vi "Test SenseHat.Actor.vi"() -> ()   [LabVIEW 2020]
uses:
  src/RPI.SenseHat.Joystick/TypeDefs/Joystick.ctl
  <vilib>/ActorFramework/Message Enqueuer/Message Enqueuer.lvclass/Message Enqueuer.ctl
  src/RPI.SenseHat.Actor/RPI.SenseHat.Actor Messages/Fill Display Msg/Fill Display Msg.lvclass/Fill Display Msg.ctl
  src/RPI.SenseHat.Actor/RPI.SenseHat.Actor Messages/Draw Display Msg/Draw Display Msg.lvclass/Draw Display Msg.ctl
  src/RPI.SenseHat.Actor/RPI.SenseHat.Actor Messages/Start Stop Joystick Msg/Start Stop Joystick Msg.lvclass/Start Stop Joystick Msg.ctl
  <vilib>/ActorFramework/Message Enqueuer/Enqueue.vi
  src/RPI.SenseHat.Actor/RPI.SenseHat.Actor Messages/Reset Display Msg/Reset Display Msg.lvclass
  C:/Program Files (x86)/National Instruments/LabVIEW 2020/vi.lib/ActorFramework/Message/Message.lvclass
  src/RPI.SenseHat.Actor/RPI.SenseHat.Actor Messages/Clear Display Msg/Clear Display Msg.lvclass
  src/RPI.SenseHat.Actor/RPI.SenseHat.Actor Messages/Fill Display Msg/Fill Display Msg.lvclass
  src/RPI.SenseHat.Actor/RPI.SenseHat.Actor Messages/Draw Display Msg/Draw Display Msg.lvclass
  src/RPI.SenseHat.Actor/RPI.SenseHat.Actor Messages/Start Stop Joystick Msg/Start Stop Joystick Msg.lvclass
  <vilib>/ActorFramework/Stop Msg/Stop Msg.lvclass
  <vilib>/ActorFramework/Message Priority Queue/Priority Enqueue.vi
  src/RPI.SenseHat.Actor/RPI.SenseHat.Actor.lvlib
  src/RPI.SenseHat.Actor/RPI.SenseHat.Actor Messages/Get RPI.Name Msg/Get Device Name Msg.lvclass
  src/RPI.SenseHat.Actor/RPI.SenseHat.Actor Messages/Get Joystick State Msg WFR/Get Joystick State Msg WFR.lvclass
  src/RPI.SenseHat.Joystick/RPI.SenseHat.Joystick.lvlib
panel:
  in  "Start?":bool
  out "Joystick":T1
  out "Front Panel Window:Title":string
  in  "Stop":bool
  in  "Image":u32[][](array[colorbox])=[[0, 16777228, 16777228, 16777228, 16777228, 16777228, 0, 0], [0, 15977803, 15977803, 15977803, 15977803, 15977803, 16777228, 0], [0, 15977803, 0, 0, 0, 0, 15977803, 0], [0, 15977803, 0, 0, 0, 0, 15977803, 0], [0, 15977803, 15977803, 15977803, 15977803, 15977803, 0, 0], [0, 15977803, 0, 0, 0, 0, 15977803, 0], [0, 15977803, 0, 0, 0, 0, 15977803, 0], [0, 15977803, 15977803, 15977803, 15977803, 15977803, 0, 16777222]]
  in  "Color":u32(colorbox)
  in  "Actions":T2(radio)=enum."reset"
  out "Error Out":errorcluster
  out "Device Name":string
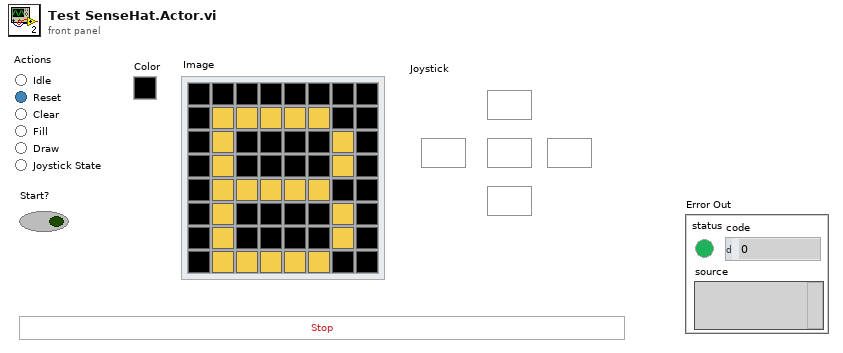
[diagram p1: front panel]
types:
  T1 = typedef "RPI.SenseHat.Joystick.lvlib/Joystick.ctl" = cluster{"Enter":bool, "Down":bool, "Up":bool, "Right":bool, "Left":bool}
  T2 = enum32{"idle", "reset", "clear", "fill", "draw", "joystick"}
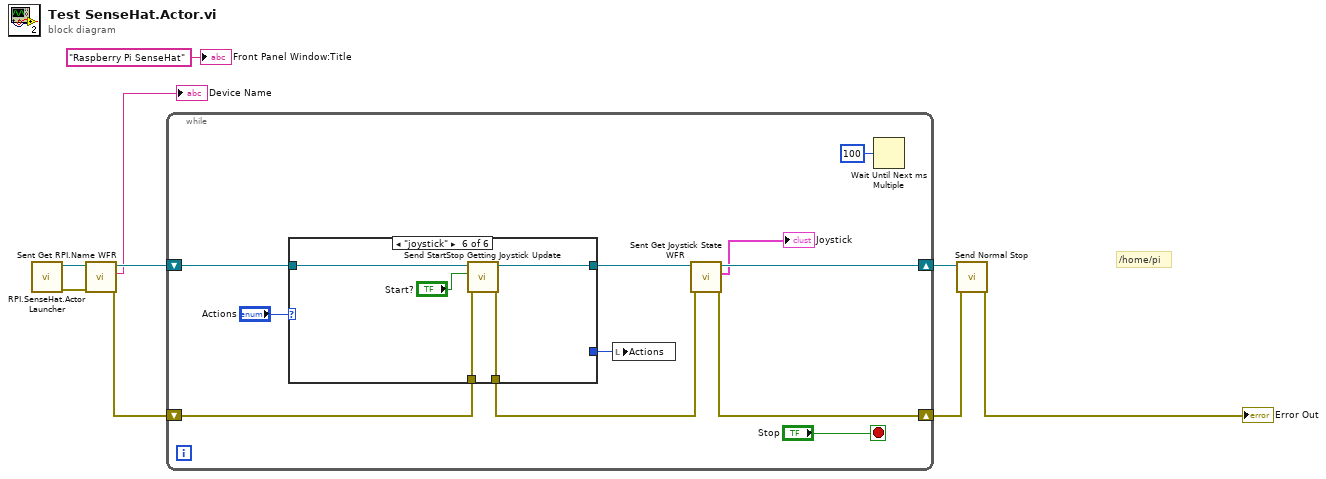
[diagram p0: block diagram]
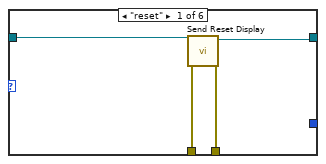
[diagram p2: hidden frame]
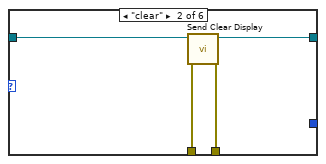
[diagram p3: hidden frame]
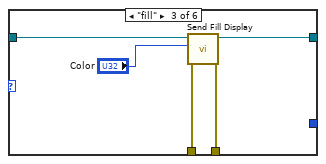
[diagram p4: hidden frame]
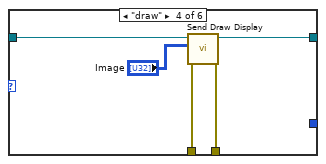
[diagram p5: hidden frame]
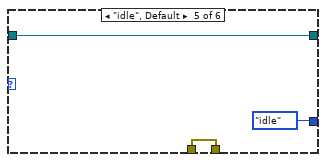
[diagram p6: hidden frame]
diagram:
  # "/home/pi"
  n1 = call "RPI.SenseHat.Actor Launcher.vi"() -> ("error out"=w7:errorcluster, "RPI.SenseHat Enqueuer"=w2:refnum<class "Message Enqueuer.lvclass">)  [unwired: 10 in]
  n2 = call "Sent Get RPI.Name WFR.vi"("error in (no error)"=w7, "Message Enqueuer"=w2) -> ("error out"=w6:errorcluster, "Reply"=→"Device Name":string, "Message Enqueuer out"=w8:refnum<class "Message Enqueuer.lvclass">)  [unwired: 7 in]
  n3 = while {
    shift-right: [w13] -> w3
    shift-left: w8 -> [w20]
    shift-right: [w10] -> w4
    shift-left: w6 -> [w19]
    stop <- "Stop" stop-if-true
    n4 = case shown="\"joystick\"" "Actions" {
      tunnel: [w21 w28 w31 w36 w41 w44] -> w11
      tunnel: w19 -> [w22 w27 w30 w35 w41 w43]
      tunnel: w20 -> [w24 w25 w33 w38 w40 w46]
      tunnel: [w23 w26 w32 w37 w40 w45] -> w14
      tunnel: [_ _ _ _ T2."idle" ("Actions") _] -> w16
      frame "reset" {
        n5 = call "Send Reset Display.vi"("error in (no error)"=w22, "Message Enqueuer"=w24) -> ("error out"=w21:errorcluster, "Message Enqueuer out"=w23:refnum<class "Message Enqueuer.lvclass">)  [unwired: 8 in]
      }
      frame "clear" {
        n6 = call "Send Clear Display.vi"("error in (no error)"=w27, "Message Enqueuer"=w25) -> ("error out"=w28:errorcluster, "Message Enqueuer out"=w26:refnum<class "Message Enqueuer.lvclass">)  [unwired: 8 in]
      }
      frame "fill" {
        n7 = call "Send Fill Display.vi"("error in (no error)"=w30, "Color"="Color", "Message Enqueuer"=w33) -> ("error out"=w31:errorcluster, "Message Enqueuer out"=w32:refnum<class "Message Enqueuer.lvclass">)  [unwired: 7 in]
      }
      frame "draw" {
        n8 = call "Send Draw Display.vi"("error in (no error)"=w35, "Color"="Image", "Message Enqueuer"=w38) -> ("error out"=w36:errorcluster, "Message Enqueuer out"=w37:refnum<class "Message Enqueuer.lvclass">)  [unwired: 7 in]
      }
      frame "idle", Default {
      }
      frame "joystick" {
        n9 = call "Send StartStop Getting Joystick Update.vi"("error in (no error)"=w43, "Start?"="Start?", "Message Enqueuer"=w46) -> ("error out"=w44:errorcluster, "Message Enqueuer out"=w45:refnum<class "Message Enqueuer.lvclass">)  [unwired: 7 in]
      }
    }
    n10 = local write "Actions"(w16) -> ()
    n11 = call "Sent Get Joystick State WFR.vi"("error in (no error)"=w11, "Message Enqueuer"=w14) -> ("error out"=w10:errorcluster, "Reply"=→"Joystick":T1, "Message Enqueuer out"=w13:refnum<class "Message Enqueuer.lvclass">)  [unwired: 7 in]
    n12 = Wait Until Next ms Multiple(millisecond multiple=u32 100) -> ()  [unwired: 1 out]
  }
  n13 = call <vilib>:"Send Normal Stop.vi"("error in (no error)"=w4, "Message Enqueuer"=w3) -> ("error out"=→"Error Out":errorcluster)  [unwired: 9 in]
  "Front Panel Window:Title" <- "Raspberry Pi SenseHat" ("Front Panel Window:Title")
